vi "clLabview_writeLVSR.vi"(0 "vi_lib.lvlib:clLabview.lvclass":refnum<class "clLabview.lvclass">, 2 "new lib Password":string) -> (7 "vi_lib.lvlib:clLabview.lvclass [Out]":refnum<class "clLabview.lvclass">)   [LabVIEW 2020, in "vi_lib.lvlib" / "clLabview.lvclass"]
uses:
  clLabview.lvclass
  clFileReader/clFileReader.lvclass
  vi_lib.lvlib
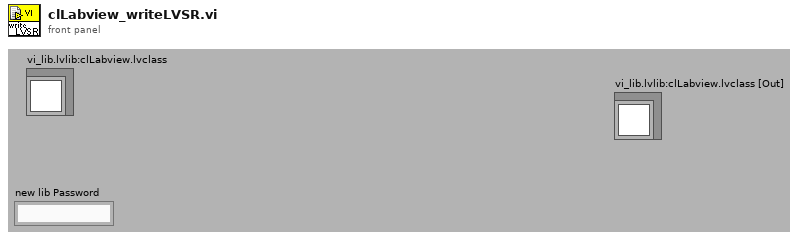
[diagram p1: front panel]
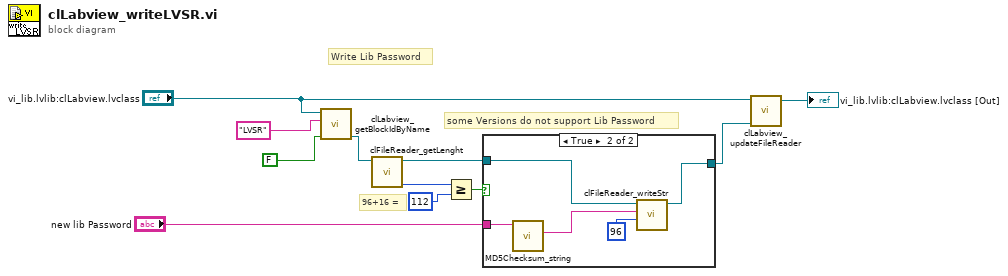
[diagram p0: block diagram]
diagram:
  # "Write Lib Password"
  # "some Versions do not support Lib Password"
  # "96+16 ="
  n1 = call "clLabview_getBlockIdByName.vi"("use compression (off)"=FALSE, "Block Name"="LVSR", "vi_lib.lvlib:clLabview.lvclass"="vi_lib.lvlib:clLabview.lvclass") -> ("Block Content"=w8:refnum<class "clFileReader.lvclass">)  [unwired: 1 in, 6 out]
  n2 = call "clFileReader_getLenght.vi"("clFileReader.lvclass IN"=w8) -> ("blocklen"=w5:u32, "clFileReader.lvclassOut"=w7:refnum<class "clFileReader.lvclass">)  [unwired: 9 out]
  n3 = Greater Or Equal?(x=w5, y=u32 112) -> (x >= y?=w6:bool)
  n4 = case shown="True" w6 {
    tunnel: w7 -> [w12 w17]
    tunnel: [w12 w15] -> w3
    tunnel: "new lib Password" -> [_ w14]
    frame False {
    }
    frame True {
      n5 = call "MD5Checksum_string.vi"("Message String"=w14) -> ("MD5 message-digest (Ascii)"=w13:string)  [unwired: 10 out]
      n6 = call "clFileReader_writeStr.vi"("offset"=u32 96, "ReadStr - IN Value"=w13, "clFileReader.lvclass IN"=w17) -> ("clFileReader.lvclass OUT"=w15:refnum<class "clFileReader.lvclass">)  [unwired: 8 out]
    }
  }
  n7 = call "clLabview_updateFileReader.vi"("clFileReader.lvclass OUT"=w3, "vi_lib.lvlib:clLabview.lvclass"="vi_lib.lvlib:clLabview.lvclass") -> ("vi_lib.lvlib:clLabview.lvclass 2"=→"vi_lib.lvlib:clLabview.lvclass [Out]":refnum<class "clLabview.lvclass">)  [unwired: 9 out]
